vi "ComparisionOps.vi"() -> ()   [LabVIEW 2019]
panel:
  out "Result":bool
  in  "a":dbl
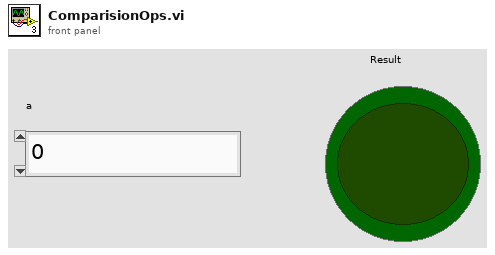
[diagram p1: front panel]
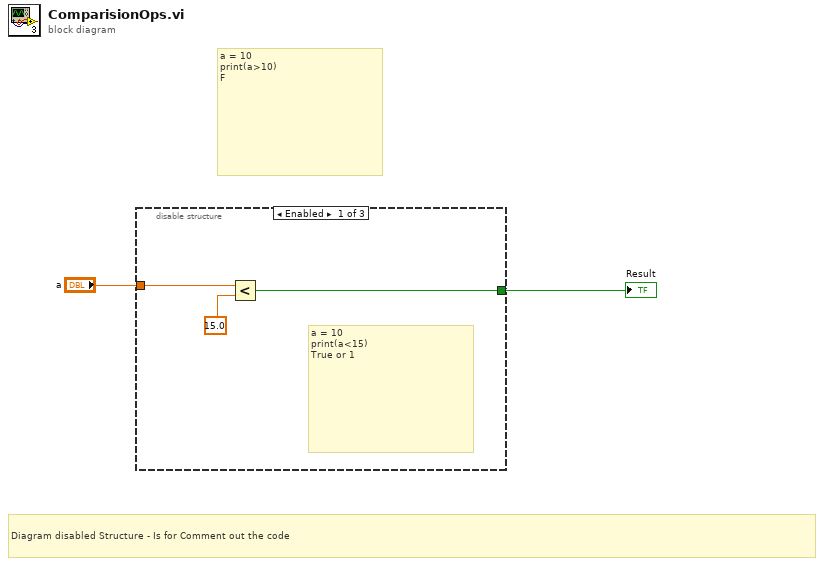
[diagram p0: block diagram]
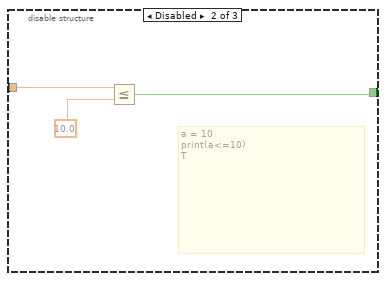
[diagram p2: hidden frame]
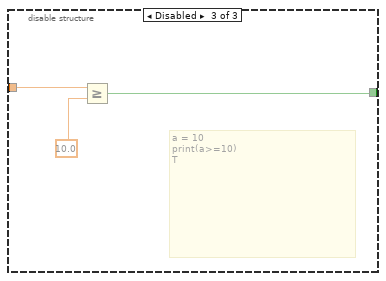
[diagram p3: hidden frame]
diagram:
  # "Diagram disabled Structure - Is for Comment out the code"
  # "a = 10\nprint(a>10)\nF"
  n1 = disable-structure shown="Enabled" {
    disable-tunnel: "a" -> [w5 w8 w11]
    disable-tunnel: [w3 w6 w9] -> w1
    frame Enabled {
      # "a = 10\nprint(a<15)\nTrue or 1"
      n2 = Less?(x=w5, y=15.0) -> (x < y?=w3:bool)
    }
    frame Disabled {
      # "a = 10\nprint(a<=10)\nT"
      n3 = Less Or Equal?(x=w8, y=10.0) -> (x <= y?=w6:bool)
    }
    frame Disabled {
      # "a = 10\nprint(a>=10)\nT"
      n4 = Greater Or Equal?(x=w11, y=10.0) -> (x >= y?=w9:bool)
    }
  }
  "Result" <- w1
